vi "MaxIterationGV.vi"(8 "error in (no error)":errorcluster, 9 "SetMaxIteration":dbl, 10 "GetOrSet":enum16{"Get", "Set"}(ring)) -> (0 "error out":errorcluster, 2 "MaxIteration":dbl)   [LabVIEW 2016]
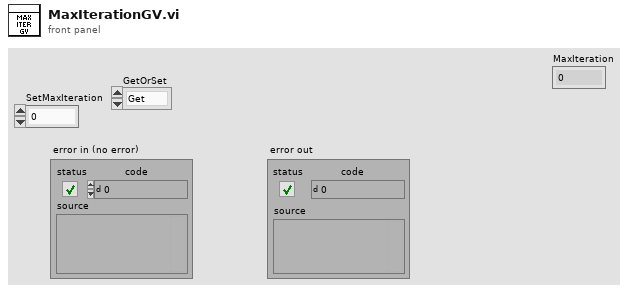
[diagram p1: front panel]
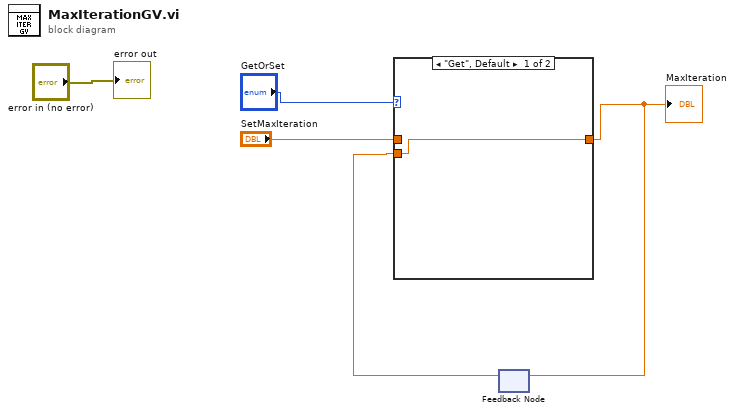
[diagram p0: block diagram]
diagram:
  n1 = feedback #1() -> (w1:dbl)  [unwired: 1 in]
  n2 = case shown="\"Get\", Default" "GetOrSet" {
    tunnel: [w6 w7] -> w2
    tunnel: "SetMaxIteration" -> [_ w7]
    tunnel: w1 -> [w6 _]
    frame "Get", Default {
    }
    frame "Set" {
    }
  }
  "MaxIteration" <- w2
  n3 = feedback-in #1(w2) -> ()
  "error out" <- "error in (no error)"
